vi "Cobra_Front_Panel_Basic.vi"() -> ()   [LabVIEW 2015]
panel:
  in  "RESET Button":bool
  in  "Internal Trigger":bool=TRUE
  in  "EXIT":bool
  in  "Line Scan Enable":bool=TRUE
  in  "Line Time Value":u16=90 step=1
  in  "Integration Time Value":u16=100 min=1 max=32767 step=1
  in  "Offset Value":u16=255 max=255 step=1
  in  "Gain Value":u16=187 max=255 step=1
  out "Configuration String Sent":string
  out "Failure":bool
  out "Initialized":bool
  in  "Set":bool
  out "Characters Read":u32
  out "IMAQ Session Out":refnum<k11>
  out "Command Data Read":string
  out "Error Output":errorcluster
  in  "error in (no error)":errorcluster
  # "Suggested Starting Values:\n\nGain: 187\nOffset: 255\nIntegration Time: 90\nLine Time: 100"
  # "Inital Setup and Connection:\n\n  1. Launch NI MAX, select the camera (should be img0).\n  2. Load the supplied *.icd file for the camera.\n  3. Close NI MAX.\n  4. Run this VI and click the \"Set all\" button."
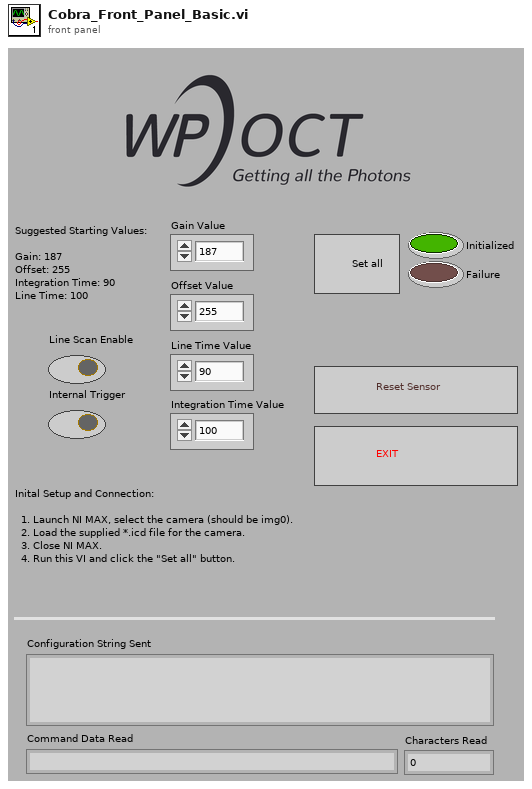
[diagram p1: front panel]
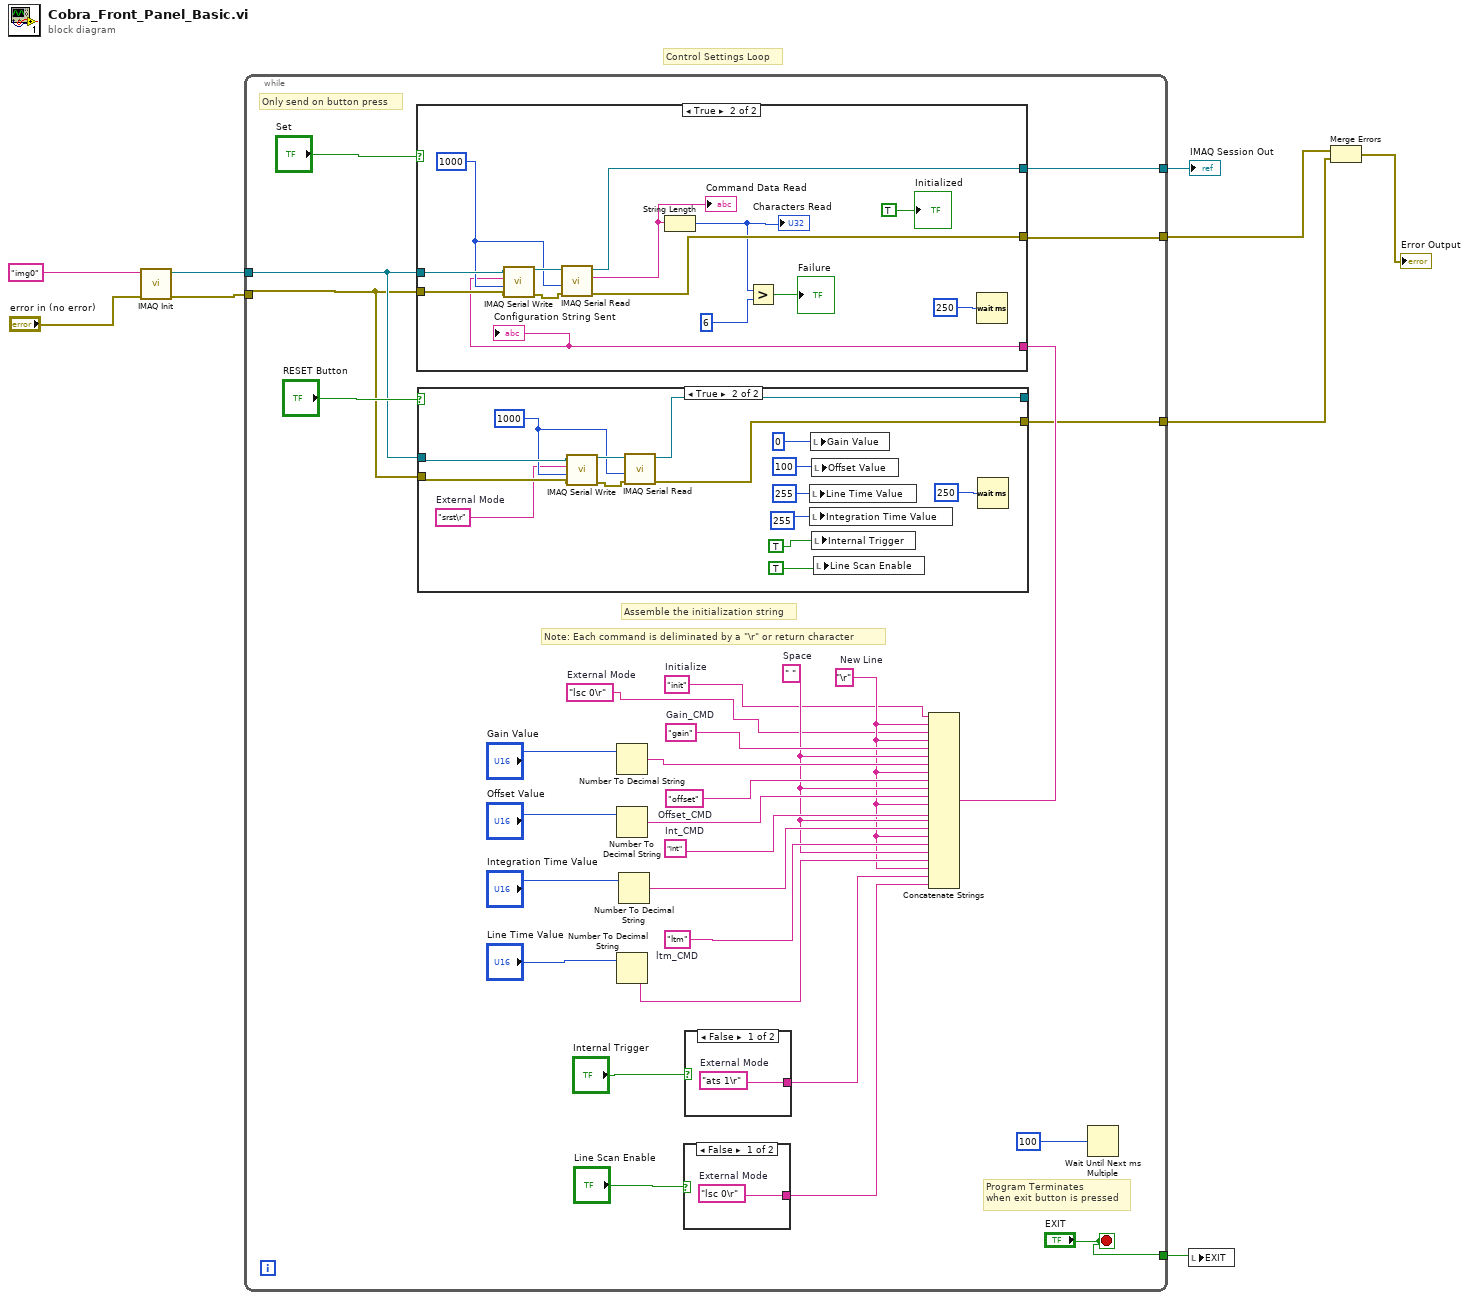
[diagram p0: block diagram]
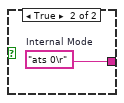
[diagram p3: hidden frame]
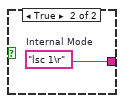
[diagram p5: hidden frame]
diagram:
  # "Control Settings Loop"
  n1 = call <vilib>:"IMAQ Init.vi"("error in (no error)"="error in (no error)", "Interface Name"="img0") -> ("error out"=w6:errorcluster, "IMAQ Session Out"=w7:refnum<k11>)  [unwired: 8 in]
  n2 = while {
    tunnel: w7 -> [w13]
    tunnel: w6 -> [w12]
    tunnel: [w39] -> w8
    tunnel: [w38] -> w5
    tunnel: [w11] -> w2
    tunnel: ["EXIT"] -> w1
    stop <- "EXIT" stop-if-true
    w19 = "lsc 0\r"  # External Mode
    w27 = "ltm"  # ltm_CMD
    w26 = "int"  # Int_CMD
    w25 = "offset"  # Offset_CMD
    w24 = "gain"  # Gain_CMD
    w21 = " "  # Space
    w20 = "\r"  # New Line
    w18 = "init"  # Initialize
    # "Program Terminates\nwhen exit button is pressed"
    # "Only send on button press"
    # "Note: Each command is deliminated by a \"\\r\" or return character"
    # "Assemble the initialization string"
    n3 = case shown="True" "RESET Button" {
      tunnel: w13 -> [w41 w51]
      tunnel: w12 -> [w40 w49]
      tunnel: [w41 w56] -> _
      tunnel: [w40 w55] -> w11
      frame False {
      }
      frame True {
        w48 = "srst\r"  # External Mode
        w50 = 1000
        n4 = call <vilib>:"IMAQ Serial Write.vi"("error in (no error)"=w49, "Timeout"=w50, "String to write"=w48, "IMAQ Session In"=w51) -> ("error out"=w52:errorcluster, "IMAQ Session Out"=w53:refnum<k11>)  [unwired: 4 in]
        n5 = call <vilib>:"IMAQ Serial Read.vi"("error in (no error)"=w52, "Timeout"=w50, "IMAQ Session In"=w53) -> ("error out"=w55:errorcluster, "IMAQ Session Out"=w56:refnum<k11>)  [unwired: 3 in, 2 out]
        n6 = local write "Line Time Value"(255) -> ()
        n7 = local write "Integration Time Value"(255) -> ()
        n8 = local write "Gain Value"(0) -> ()
        n9 = local write "Offset Value"(100) -> ()
        n10 = local write "Internal Trigger"(TRUE) -> ()
        n11 = local write "Line Scan Enable"(TRUE) -> ()
        n12 = Wait (ms)(milliseconds to wait=250) -> ()  [unwired: 1 out]
      }
    }
    n13 = Number To Decimal String(number="Gain Value") -> (decimal integer string=w28:string)  [unwired: 1 in]
    n14 = Number To Decimal String(number="Offset Value") -> (decimal integer string=w30:string)  [unwired: 1 in]
    n15 = Number To Decimal String(number="Line Time Value") -> (decimal integer string=w35:string)  [unwired: 1 in]
    n16 = Number To Decimal String(number="Integration Time Value") -> (decimal integer string=w33:string)  [unwired: 1 in]
    n17 = case shown="False" "Line Scan Enable" {
      tunnel: [w75 w76] -> w15
      frame False {
        w75 = "lsc 0\r"  # External Mode
      }
      frame True {
        w76 = "lsc 1\r"  # Internal Mode
      }
    }
    n18 = case shown="False" "Internal Trigger" {
      tunnel: [w57 w58] -> w16
      frame False {
        w57 = "ats 1\r"  # External Mode
      }
      frame True {
        w58 = "ats 0\r"  # Internal Mode
      }
    }
    n19 = Concatenate Strings(w18, w20, w19, w20, w24, w21, w28, w20, w25, w21, w30, w20, w26, w21, w33, w20, w27, w21, w35, w20, w16, w15) -> (w23:string)
    n20 = case shown="True" "Set" {
      tunnel: w13 -> [w60 w68]
      tunnel: w12 -> [w59 w66]
      tunnel: [w60 w74] -> w39
      tunnel: [w59 w73] -> w38
      tunnel: w23 -> [_ w65]
      frame False {
      }
      frame True {
        w67 = 1000
        n21 = call <vilib>:"IMAQ Serial Write.vi"("error in (no error)"=w66, "Timeout"=w67, "String to write"=w65, "IMAQ Session In"=w68) -> ("error out"=w69:errorcluster, "IMAQ Session Out"=w70:refnum<k11>)  [unwired: 4 in]
        n22 = call <vilib>:"IMAQ Serial Read.vi"("error in (no error)"=w69, "Timeout"=w67, "IMAQ Session In"=w70) -> ("error out"=w73:errorcluster, "String Read"=w64:string, "IMAQ Session Out"=w74:refnum<k11>)  [unwired: 3 in, 1 out]
        "Command Data Read" <- w64
        n23 = String Length(string=w64) -> (length=w63:i32)
        "Characters Read" <- w63
        n24 = Greater?(x=w63, y=6) -> (0:→"Failure":bool)
        n25 = Wait (ms)(milliseconds to wait=250) -> ()  [unwired: 1 out]
        "Configuration String Sent" <- w65
        "Initialized" <- TRUE
      }
    }
    n26 = Wait Until Next ms Multiple(millisecond multiple=100) -> ()  [unwired: 1 out]
  }
  "IMAQ Session Out" <- w8
  n27 = local write "EXIT"(w1) -> ()
  n28 = Merge Errors(w5, w2) -> (→"Error Output":errorcluster)
